vi "CalcDesiredVelVector_SpaceMouse_Input.vi"(8 "error in (no error)":errorcluster, 10 "Desired Speed(Throttle)":dbl) -> (0 "error IO":errorcluster)   [LabVIEW 2013]
uses:
  Controls/SpaceMouse_FilteredInput.ctl
  <vilib>/Analysis/_algsub.llb/Real Vector Norm.vi
  <vilib>/Analysis/NI_AALPro.lvlib
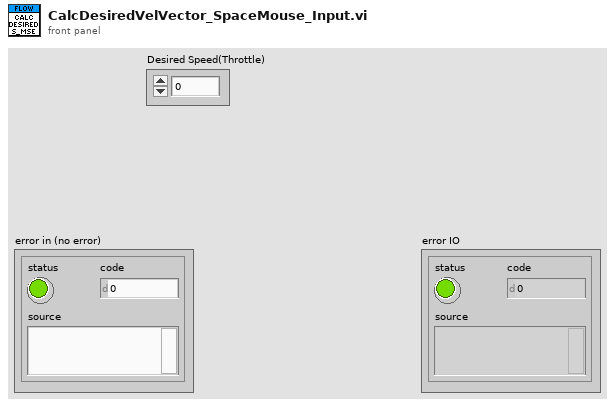
[diagram p1: front panel]
types:
  T1 = typedef "SpaceMouse_FilteredInput.ctl" = cluster{"X":dbl, "Y":dbl, "Z":dbl, "phi":dbl, "theta":dbl, "psi":dbl}
  T2 = cluster{"u_B_des":dbl, "v_B_des":dbl, "w_B_des":dbl}
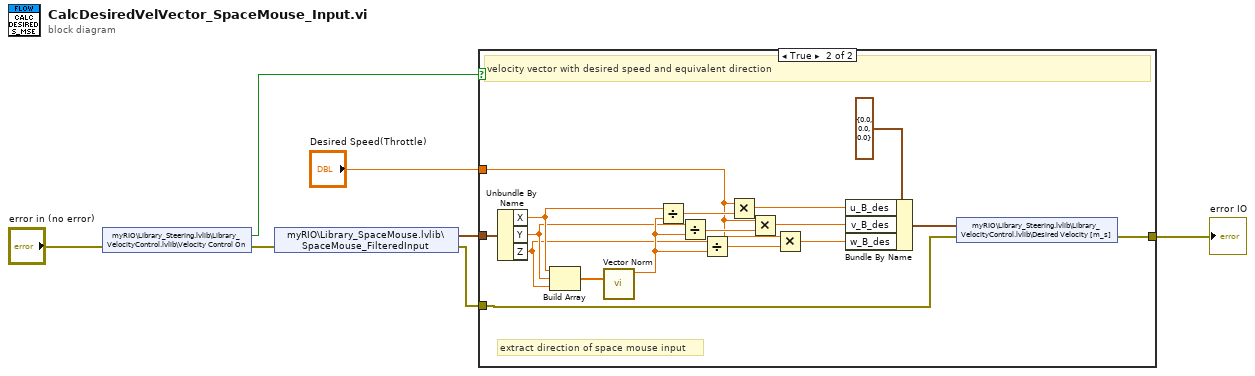
[diagram p0: block diagram]
diagram:
  n1 = shared-variable "myRIO\\Library_Steering.lvlib\\Library_VelocityControl.lvlib\\Velocity Control On"(error in="error in (no error)") -> (w7:bool, error out=w2:errorcluster)
  n2 = shared-variable "myRIO\\Library_SpaceMouse.lvlib\\SpaceMouse_FilteredInput"(error in=w2) -> (w4:T1, error out=w3:errorcluster)
  n3 = case shown="True" w7 {
    tunnel: [w8 w23] -> w6
    tunnel: w4 -> [_ w22]
    tunnel: w3 -> [w8 w21]
    tunnel: "Desired Speed(Throttle)" -> [_ w9]
    frame False {
    }
    frame True {
      # "extract direction of space mouse input"
      # "velocity vector with desired speed and equivalent direction"
      n4 = Unbundle By Name(w22) -> ("X"=w18:dbl, "Y"=w17:dbl, "Z"=w16:dbl)
      n5 = Build Array(w18, w17, w16) -> (w20:dbl[])
      n6 = call-poly <vilib>:"Vector Norm.vi"("Input Vector"=w20) -> ("norm"=w19:dbl)  [unwired: 9 in, 1 out]
      n7 = Divide(x=w18, y=w19) -> (x/y=w15:dbl)
      n8 = Divide(x=w17, y=w19) -> (x/y=w14:dbl)
      n9 = Divide(x=w16, y=w19) -> (x/y=w13:dbl)
      n10 = Multiply(x=w9, y=w15) -> (x*y=w10:dbl)
      n11 = Multiply(x=w9, y=w14) -> (x*y=w11:dbl)
      n12 = Multiply(x=w9, y=w13) -> (x*y=w12:dbl)
      n13 = Bundle By Name(cluster=T2 {"u_B_des"=0.0, "v_B_des"=0.0, "w_B_des"=0.0} ("New desired Velocity"), "u_B_des"=w10, "v_B_des"=w11, "w_B_des"=w12) -> (w24:T2)
      n14 = shared-variable "myRIO\\Library_Steering.lvlib\\Library_VelocityControl.lvlib\\Desired Velocity [m_s]"(w24, error in=w21) -> (error out=w23:errorcluster)
    }
  }
  "error IO" <- w6
